vi "test lvjson.vi"(8 "error in (no error)":errorcluster) -> (0 "error out":errorcluster)   [LabVIEW 2019, in "labview_json_tests.lvlib"]
uses:
  labview_json_tests.lvlib
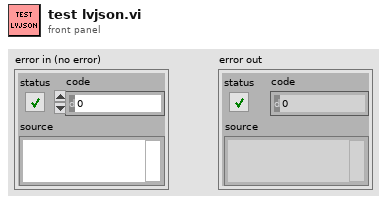
[diagram p1: front panel]
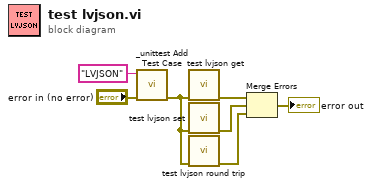
[diagram p0: block diagram]
diagram:
  n1 = call "_unittest Add Test Case.vi"("error in (no error)"="error in (no error)", "Test Case"="LVJSON") -> ("error out"=w2:errorcluster)  [unwired: 9 in]
  n2 = call "test lvjson get.vi"("error in (no error)"=w2) -> ("error out"=w4:errorcluster)  [unwired: 10 in]
  n3 = call "test lvjson set.vi"("error in (no error)"=w2) -> ("error out"=w3:errorcluster)  [unwired: 10 in]
  n4 = call "test lvjson round trip.vi"("error in (no error)"=w2) -> ("error out"=w1:errorcluster)  [unwired: 10 in]
  n5 = Merge Errors(w4, w3, w1) -> (→"error out":errorcluster)
